vi "ScalingFactors.vi"(1 "Input measurements":dbl[](array[numeric])) -> (0 "Output measurements":dbl[](array[numeric]))   [LabVIEW 2013]
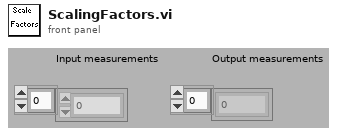
[diagram p1: front panel]
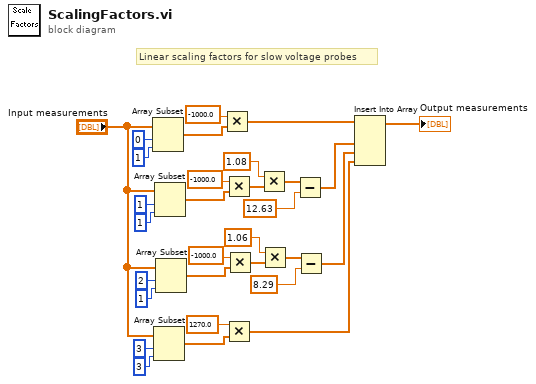
[diagram p0: block diagram]
diagram:
  # "Linear scaling factors for slow voltage probes"
  n1 = Array Subset(array="Input measurements", index=0, length=1) -> (w28:dbl[])
  n2 = Array Subset(array="Input measurements", index=3, length=3) -> (w30:dbl[])
  n3 = Array Subset(array="Input measurements", index=1, length=1) -> (w19:dbl[])
  n4 = Array Subset(array="Input measurements", index=2, length=1) -> (w11:dbl[])
  n5 = Multiply(x=-1000.0, y=w28) -> (x*y=w6:dbl[])
  n6 = Multiply(x=-1000.0, y=w19) -> (x*y=w18:dbl[])
  n7 = Multiply(x=1270.0, y=w30) -> (x*y=w3:dbl[])
  n8 = Multiply(x=-1000.0, y=w11) -> (x*y=w10:dbl[])
  n9 = Multiply(x=1.08, y=w18) -> (x*y=w16:dbl[])
  n10 = Multiply(x=1.06, y=w10) -> (x*y=w9:dbl[])
  n11 = Subtract(x=w16, y=12.63 ("x")) -> (x-y=w5:dbl[])
  n12 = Subtract(x=w9, y=8.29 ("x")) -> (x-y=w4:dbl[])
  n13 = Insert Into Array(array=w6, new element #1=w5, new element #2=w4, new element #3=w3) -> (→"Output measurements":dbl[])  [unwired: 1 in]
